vi "Robot Global Data.vi"() -> ()   [LabVIEW 2019]
doc: "This global VI can contain as many global variables as you need. Place a control on the panel, give it a good name. To read or write to it from a VI, drag the icon to the diagram of that VI. You can also drag from the project. Click on the node to change which global you access. You shouldn't have multiple locations writing to a global or it will cause a race-condition."
uses:
  <vilib>/Rock Robotics/WPI/Camera/WPI_CameraImageSize.ctl
  <vilib>/Rock Robotics/WPI/DriverStation/WPI_DriverStationRobotMode2.ctl
panel:
  out "conveyorSensor04":bool
  out "siRight":dbl
  out "siLeft":dbl
  out "intakePivotMotorActualValue":dbl
  out "conveyorMotorOutput":dbl
  out "servoOut":bool
  out "servoDown":bool
  out "servoUp":bool
  out "shooterEncoderDistance":dbl
  out "servoAngle":dbl
  out "rightEncoderInches":dbl
  out "leftEncoderInches":dbl
  out "manualShooterAngleUp":bool
  out "manualShooterAngleDown":bool
  out "shooterAnglePreset01":bool
  out "shooterAnglePreset04":bool
  out "shooterAnglePreset02":bool
  out "shooterAnglePreset03":bool
  out "shooterMotorWantedAngle":dbl
  out "shooterMotorActualAngle":dbl
  out "shooterMotorStartValue":dbl
  in  "shootCounter":i32
  out "desiredShoot":i32
  out "limeLightAim":bool
  out "limeLightOn":bool
  out "elevatorAllUp":bool
  out "pov270":bool
  out "pov90":bool
  out "elevatorAllDown":bool
  out "bottomLimit02":bool
  out "bottomLimit01":bool
  out "conveyorSensor03":bool
  in  "whichRobot?":T1=enum."andy"
  out "conveyorSensor02":bool
  out "conveyorSensor01":bool
  out "motionProfilingComplete":bool
  out "runMotionProfiling":bool
  out "rightEncoder":dbl
  out "leftEncoder":dbl
  out "rightEncoderInital":dbl
  out "leftEncoderInital":dbl
  out "intakePivotMotorWantedAngle":dbl
  out "intakePivotMotorActualAngle":dbl
  out "intakePivotMotorStartValue":dbl
  out "upperLimit02":bool
  out "upperLimit01":bool
  out "Fast Mode":bool
  out "Slow Mode":bool
  out "Drive Joystick Right Y":dbl
  out "Drive Joystick Left Y":dbl
  out "horizontalConveyorMotorToggle":bool
  out "verticalConveyorUp":bool
  out "shooter":bool
  out "verticalConveyorDown":bool
  out "manualElevatorUp/Down":dbl
  out "Joystick Right X":dbl
  out "manualIntakeUp/Down":dbl
  out "Joystick Left X":dbl
  out "intakeOut":bool
  out "intakeIn":bool
  in  "Robot Mode":T2
  in  "image size":T3=enum."320x240"
  in  "Enable Vision":bool
  # "Drive Controller"
  # "Aux Controller"
  # "Shooter Counter"
  # "Intake Motor Angle Stuff"
  # "Elevator Limit Switches"
  # "Motion Profiling"
  # "Conveyor IR Sensors"
  # "Drive Motors Encoder Values"
  # "Servo"
  # "Shooter Encoder Values"
  # "Which Robot?"
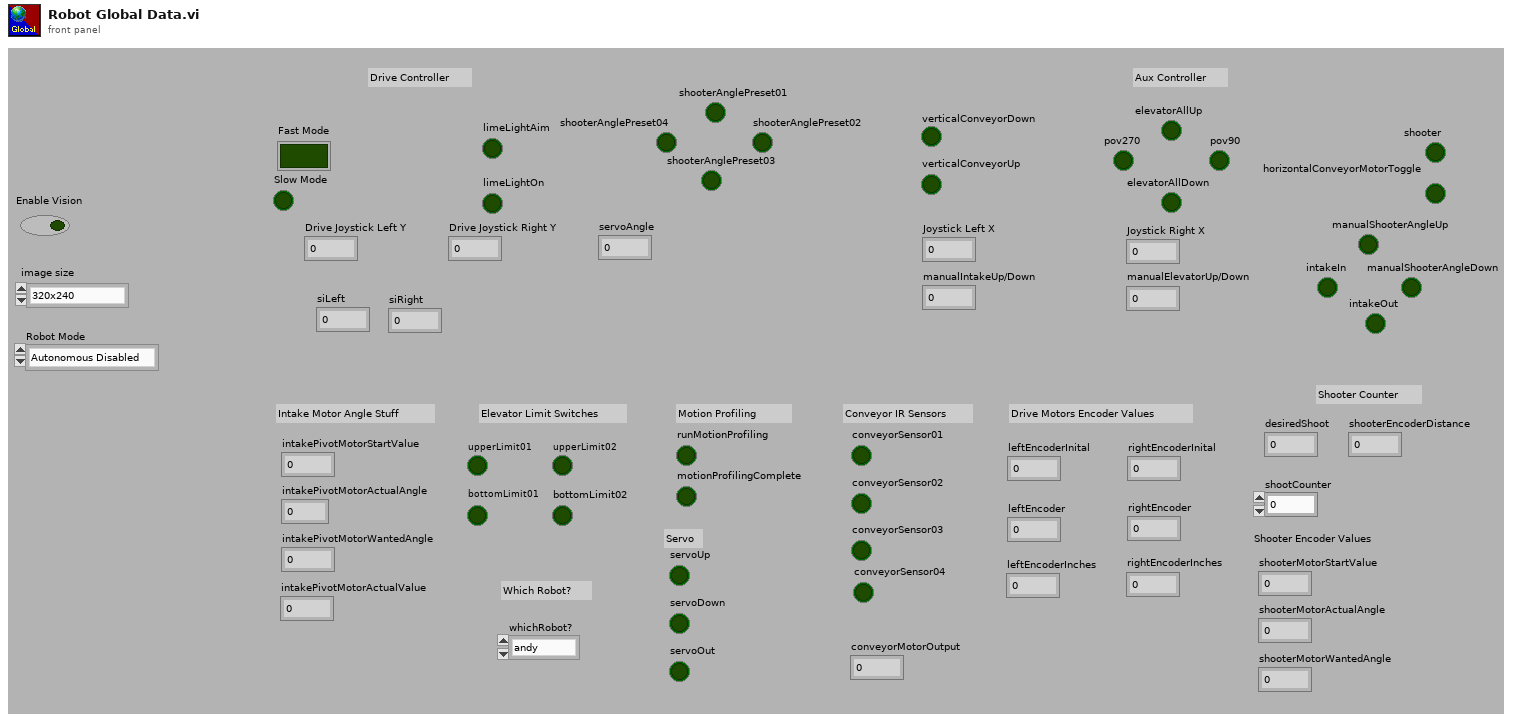
[diagram p1: front panel]
types:
  T1 = typedef "whichRobot" = enum16{"codingBot", "competitionBot", "andy"}
  T2 = typedef "WPI_DriverStationRobotMode2.ctl" = enum16{"Autonomous Disabled", "Autonomous Enabled", "Teleop Disabled", "Teleop Enabled", "Disconnected", "Finish", "Test Disabled", "Test Enabled", "Emergency Stopped"}
  T3 = typedef "WPI_CameraImageSize.ctl" = enum16{"640x480", "320x240", "160x120", "Custom"}
diagram:
